vi "Arm Auto.vi"(6 "Time":dbl, 7 "U=T\nD=F":bool, 11 "error in":errorcluster) -> (3 "error out":errorcluster)   [LabVIEW 2015]
uses:
  References/Refnums.vi
  <vilib>/ptbypt/NI_PtbyPt.lvlib
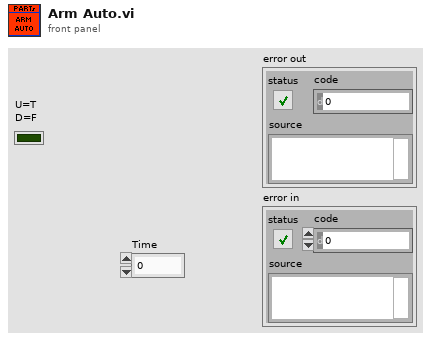
[diagram p1: front panel]
types:
  T1 = typedef "WPI_MotorControlDeviceRef.ctl" = cluster{"DeviceStatus":errorcluster, "Type":T2, "PWM":cluster{"PWM Channel":T3, "DeadBand":T4}, "CAN":cluster{"Device Number":u8, "Control Mode":T5, "Semaphore":T6, "Max Vout":dbl, "TalonSRX Control Mode":T7}, "Invert":bool}
  T2 = typedef "WPI_MotorControlType.ctl" = enum16{"PWM", "CAN", "CANTalonSRX"}
  T3 = typedef "FPGA_DIOPWMChannel.ctl" = enum8{"PWM 0", "PWM 1", "PWM 2", "PWM 3", "PWM 4", "PWM 5", "PWM 6", "PWM 7", "PWM 8", "PWM 9", "PWM MXP 0", "PWM MXP 1", "PWM MXP 2", "PWM MXP 3", "PWM MXP 4", "PWM MXP 5", "PWM MXP 6", "PWM MXP 7", "PWM MXP 8", "PWM MXP 9", "Invalid"}
  T4 = typedef "WPI_PWMDeadband.ctl" = cluster{"Name":string, "maxPositivePwm":i32, "minPositivePwm":i32, "centerPwm":i32, "maxNegativePwm":i32, "minNegativePwm":i32, "angularRange":u16}
  T5 = typedef "WPI_CANJaguar_ControlMode.ctl" = enum8{"Percent VBus", "Current", "Speed", "Position", "Voltage"}
  T6 = typedef "Semaphore RefNum" = refnum<k1>
  T7 = typedef "WPI_CANTalonSRX_APIControlMode.ctl" = enum8{"Percent VBus", "Speed", "Position", "Slave", "Unchanged / Invalid", "Voltage Compensation", "Current", "Motion Profile"}
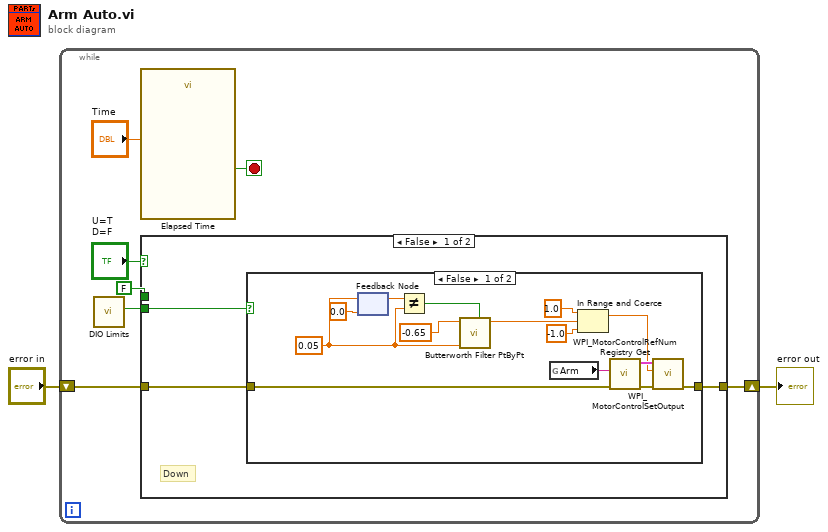
[diagram p0: block diagram]
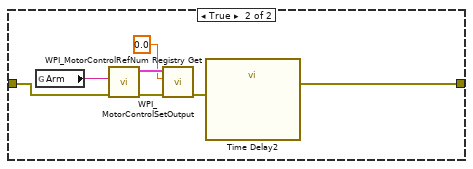
[diagram p2: hidden frame]
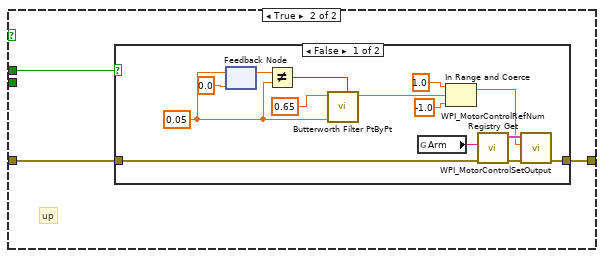
[diagram p3: hidden frame]
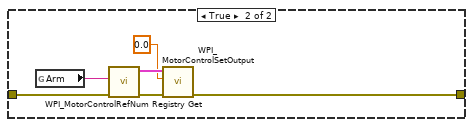
[diagram p4: hidden frame]
diagram:
  n1 = while {
    shift-right: [w8] -> w1
    shift-left: "error in" -> [w9]
    stop <- w5 stop-if-true
    n2 = call "DIO Limits.vi"() -> ("Bottom Limit"=w7:bool)  [unwired: 10 in, 1 out]
    n3 = call "Elapsed Time"("Set Start Time (s)"="Time") -> ("Time has Elapsed"=w5:bool)  [unwired: 11 in, 7 out]
    n4 = case shown="False" "U=T\nD=F" {
      tunnel: w9 -> [w12 w36]
      tunnel: [w11 w34] -> w8
      tunnel: w7 -> [w10 _]
      tunnel: FALSE ("Top Limit") -> [_ w35]
      frame False {
        # "Down"
        n5 = case shown="False" w10 {
          tunnel: w12 -> [w15 w29]
          tunnel: [w13 w27] -> w11
          frame False {
            w23 = 0.05 ("Low Pass Filter Average Length")
            n6 = feedback #1(0.0 ("Low Pass Filter Average Length")) -> (w20:dbl)
            n7 = feedback-in #1(w23) -> ()
            n8 = Not Equal?(x=w20, y=w23) -> (x != y?=w21:bool)
            n9 = call <vilib>:"Butterworth Filter PtByPt.vi"("initialize"=w21, "low cutoff freq: fl"=w23, "x"=-0.65) -> ("Filtered x"=w17:dbl)  [unwired: 6 in, 1 out]
            n10 = global read "Refnums.vi" "Arm"() -> (w26:string)
            n11 = In Range and Coerce(upper limit=1.0, x=w17, lower limit=-1.0) -> (coerced(x)=w16:dbl)  [unwired: 1 out]
            n12 = call <vilib>:"WPI_MotorControlRefNum Registry Get.vi"("error in (no error)"=w15, "refnum name"=w26) -> ("error out"=w24:errorcluster, "MotorControlDevRef"=w25:T1)  [unwired: 8 in]
            n13 = call <vilib>:"WPI_MotorControlSetOutput.vi"("error in (no error)"=w24, "Output"=w16, "MotorControlDevRef"=w25) -> ("error out"=w13:errorcluster)  [unwired: 6 in, 2 out]
          }
          frame True {
            n14 = global read "Refnums.vi" "Arm"() -> (w33:string)
            n15 = call <vilib>:"WPI_MotorControlRefNum Registry Get.vi"("error in (no error)"=w29, "refnum name"=w33) -> ("error out"=w31:errorcluster, "MotorControlDevRef"=w32:T1)  [unwired: 8 in]
            n16 = call <vilib>:"WPI_MotorControlSetOutput.vi"("error in (no error)"=w31, "Output"=0.0, "MotorControlDevRef"=w32) -> ("error out"=w28:errorcluster)  [unwired: 6 in, 2 out]
            n17 = call "Time Delay2"("error in (no error)"=w28) -> ("error out"=w27:errorcluster)  [unwired: 10 in]
          }
        }
      }
      frame True {
        # "up"
        n18 = case shown="False" w35 {
          tunnel: w36 -> [w39 w52]
          tunnel: [w37 w51] -> w34
          frame False {
            w47 = 0.05 ("Low Pass Filter Average Length")
            n19 = feedback #2(0.0 ("Low Pass Filter Average Length")) -> (w44:dbl)
            n20 = feedback-in #2(w47) -> ()
            n21 = Not Equal?(x=w44, y=w47) -> (x != y?=w45:bool)
            n22 = call <vilib>:"Butterworth Filter PtByPt.vi"("initialize"=w45, "low cutoff freq: fl"=w47, "x"=0.65) -> ("Filtered x"=w41:dbl)  [unwired: 6 in, 1 out]
            n23 = global read "Refnums.vi" "Arm"() -> (w50:string)
            n24 = In Range and Coerce(upper limit=1.0, x=w41, lower limit=-1.0) -> (coerced(x)=w40:dbl)  [unwired: 1 out]
            n25 = call <vilib>:"WPI_MotorControlRefNum Registry Get.vi"("error in (no error)"=w39, "refnum name"=w50) -> ("error out"=w48:errorcluster, "MotorControlDevRef"=w49:T1)  [unwired: 8 in]
            n26 = call <vilib>:"WPI_MotorControlSetOutput.vi"("error in (no error)"=w48, "Output"=w40, "MotorControlDevRef"=w49) -> ("error out"=w37:errorcluster)  [unwired: 6 in, 2 out]
          }
          frame True {
            n27 = global read "Refnums.vi" "Arm"() -> (w56:string)
            n28 = call <vilib>:"WPI_MotorControlRefNum Registry Get.vi"("error in (no error)"=w52, "refnum name"=w56) -> ("error out"=w54:errorcluster, "MotorControlDevRef"=w55:T1)  [unwired: 8 in]
            n29 = call <vilib>:"WPI_MotorControlSetOutput.vi"("error in (no error)"=w54, "Output"=0.0, "MotorControlDevRef"=w55) -> ("error out"=w51:errorcluster)  [unwired: 6 in, 2 out]
          }
        }
      }
    }
  }
  "error out" <- w1
